vi "Calculate Code Transitions - Sine.vi"(9 "midpoint offset":dbl, 10 "estimated amplitude (pk-pk)":dbl, 11 "histogram":i32[](array[numeric])) -> (2 "codes":i32[](array[numeric]), 3 "code transitions":dbl[](array[numeric]))   [LabVIEW 2021]
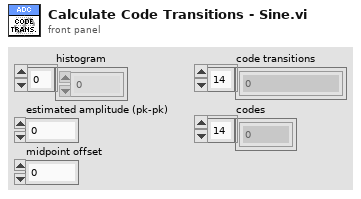
[diagram p1: front panel]
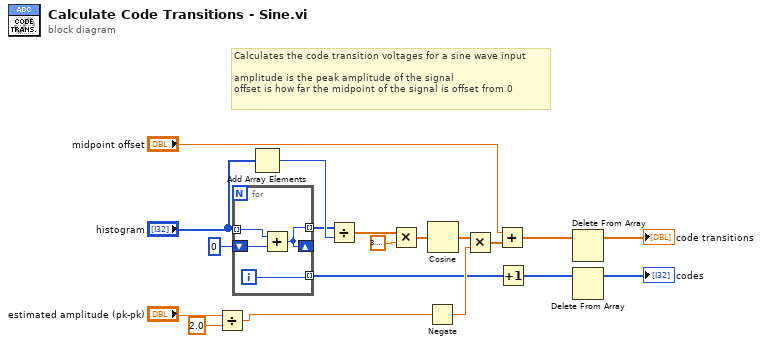
[diagram p0: block diagram]
diagram:
  # "Calculates the code transition voltages for a sine wave input\n\namplitude is the peak amplitude of the signal\noffset is how far the midpoint of the signal is offset from 0"
  n1 = Divide(x="estimated amplitude (pk-pk)", y=2.0) -> (x/y=w7:dbl)
  n2 = for {
    tunnel: "histogram" -> [w22] mode=indexing
    shift-right: [w21] -> _
    shift-left: 0 -> [w23]
    tunnel: [w21] -> w10 mode=indexing
    tunnel: [w20] -> w5 mode=indexing
    i -> [w20]
    n3 = Add(x=w22, y=w23) -> (x+y=w21:i32)
  }
  n4 = Add Array Elements(numeric array="histogram") -> (sum=w19:i32)
  n5 = Divide(x=w10, y=w19) -> (x/y=w11:dbl[])
  n6 = Multiply(x=w11, y=3.141592653589793) -> (x*y=w13:dbl[])
  n7 = Negate(x=w7) -> (-x=w15:dbl)
  n8 = Cosine(x=w13) -> (cos(x)=w14:dbl[])
  n9 = Multiply(x=w14, y=w15) -> (x*y=w16:dbl[])
  n10 = Add(x="midpoint offset", y=w16) -> (x+y=w4:dbl[])
  n11 = Increment(x=w5) -> (x+1=w2:i32[])
  n12 = Delete From Array(array=w4) -> (array with subset deleted=→"code transitions":dbl[])  [unwired: 2 in, 1 out]
  n13 = Delete From Array(array=w2) -> (array with subset deleted=→"codes":i32[])  [unwired: 2 in, 1 out]
